vi "Set Home Impl.vi"(8 "error in (no error)":errorcluster, 11 "Virtual Stage in":refnum<class "Simulated Stage.lvclass">) -> (0 "error out":errorcluster, 3 "Virtual Stage out":refnum<class "Simulated Stage.lvclass">)   [LabVIEW 2023, in "Simulated Stage.lvlib" / "Simulated Stage.lvclass"]
uses:
  Simulated Stage.lvclass
  Simulated Stage.lvclass/Simulated Stage.ctl
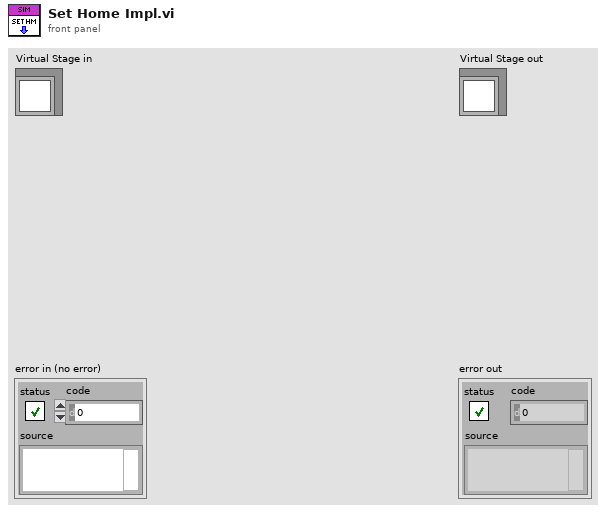
[diagram p1: front panel]
types:
  T1 = typedef "Stage Position.ctl" = cluster{"X (mm)":dbl, "Y (mm)":dbl, "Z (mm)":dbl}
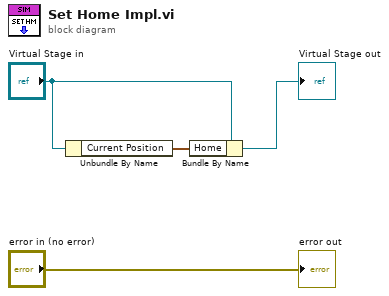
[diagram p0: block diagram]
diagram:
  n1 = Unbundle By Name("Virtual Stage in") -> ("Current Position"=w1:T1)
  n2 = Bundle By Name(cluster="Virtual Stage in", "Home"=w1) -> (→"Virtual Stage out":refnum<class "Simulated Stage.lvclass">)
  "error out" <- "error in (no error)"
